vi "calculateDelta.vi"(8 "error in (no error)":errorcluster, 11 "GuassianNoiseWave in":refnum<class "GuassianNoiseWave.lvclass">) -> (0 "error out":errorcluster, 2 "Delta Timestamp":dbl format="%.9f", 3 "GuassianNoiseWave out":refnum<class "GuassianNoiseWave.lvclass">)   [LabVIEW 2015, in "GuassianNoiseWave.lvclass"]
uses:
  GuassianNoiseWave.lvclass
  GuassianNoiseWave.lvclass/GuassianNoiseWave.ctl
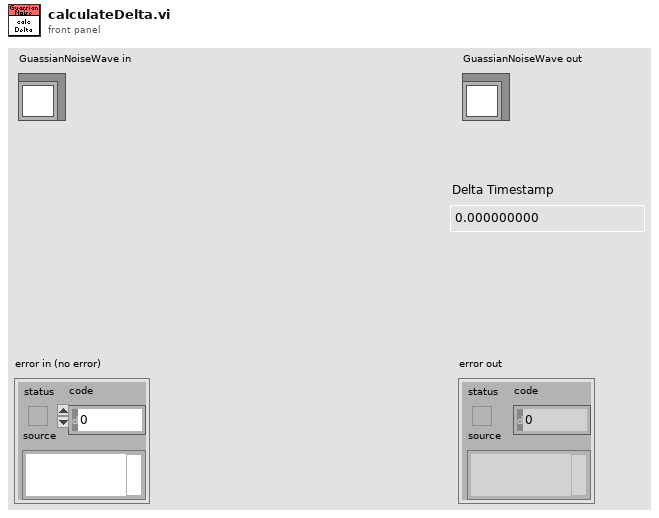
[diagram p1: front panel]
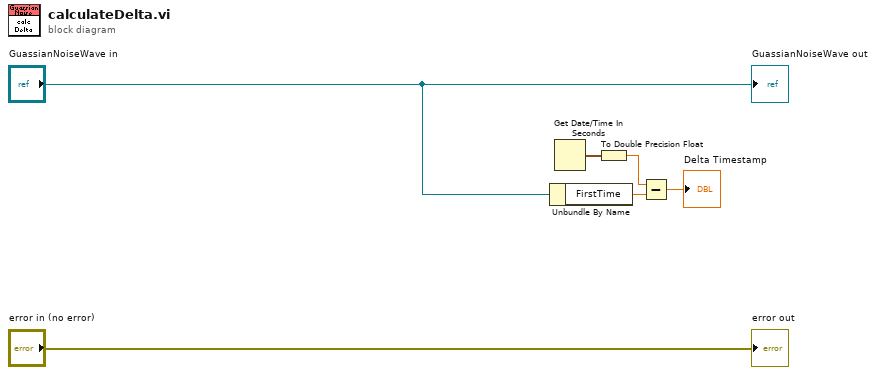
[diagram p0: block diagram]
diagram:
  n1 = Unbundle By Name("GuassianNoiseWave in") -> ("FirstTime"=w4:dbl)
  n2 = Get Date/Time In Seconds() -> (seconds since 1Jan1904=w2:timestamp)
  n3 = To Double Precision Float(number=w2) -> (double precision float=w5:dbl)
  n4 = Subtract(x=w5, y=w4) -> (x-y=→"Delta Timestamp":dbl)
  "error out" <- "error in (no error)"
  "GuassianNoiseWave out" <- "GuassianNoiseWave in"
